vi "mod2.vi"() -> ()   [LabVIEW 2016]
doc: "\"Discrete LED demo.vi\" -- Demonstrate a discrete LED connected to a digital output.\n\nInstructions:\n\n-- Click the 'enable blinker' button to toggle between blinking mode\nand static mode.\n-- In static mode, click the 'digital level' button to set the state of the\ndigital output.\n-- The 'digital output state' LED indicator shows the state of the\ndigital output (on = high, off = low)."
uses:
  <vilib>/myRIO/Common/Instrument Driver Framework/myRIO v1.0/UART/vis/myRIO v1.0 Close UART.vi
  <vilib>/Utility/error.llb/Error Cluster From Error Code.vi
  <vilib>/myRIO/Common/Instrument Driver Framework/myRIO v1.0/DIO/vis/myRIO v1.0 Write DIO.vi
  <vilib>/myRIO/Common/Instrument Driver Framework/Utilities/vis/FPGA Ref Manager.vi
  <vilib>/myRIO/Common/Instrument Driver Framework/myRIO v1.0/myRIO v1.0 Reset FPGA.vi
  <vilib>/myRIO/Common/Instrument Driver Framework/myRIO v1.0/IRQ/vis/myRIO v1.0 IRQ Info FGV.vi
  <vilib>/myRIO/Common/Instrument Driver Framework/myRIO v1.0/IRQ/vis/myRIO v1.0 Timer IRQ Info FGV.vi
  <vilib>/myRIO/Common/Instrument Driver Framework/myRIO v1.0/IRQ/vis/myRIO v1.0 ISR Agent.vi
  <vilib>/myRIO/Instrument Drivers/Utilities/Utilities.lvlib
  <vilib>/myRIO/Instrument Drivers/Onboard IO/DIO/DIO.lvlib
panel:
  in  "String":string
  out "error out":errorcluster
  in  "error in (no error)":errorcluster
  in  "[ESC]":bool
  # "7-Segment LED demo"
  # "segment 'a'"
  # "segment 'b'"
  # "segment 'c'"
  # "segment 'd'"
  # "segment 'e'"
  # "segment 'f'"
  # "segment 'g'"
  # "decimal point"
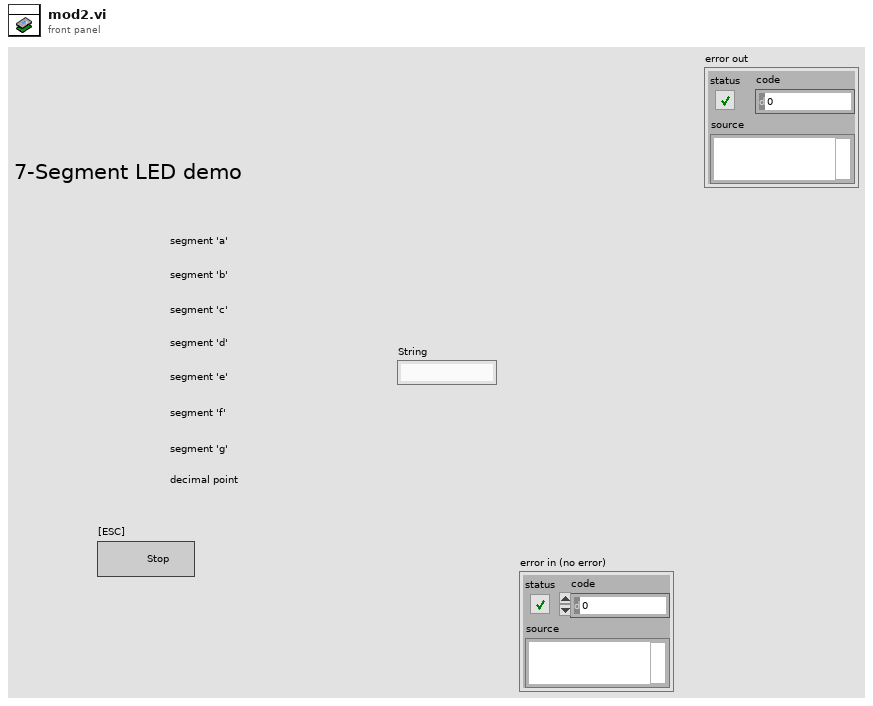
[diagram p1: front panel]
types:
  T1 = typedef "DIO.lvlib/DIO Reference.ctl" = cluster{"myRIO Reference":T2, "DIO Channels List":T6}
  T2 = typedef "myRIO Generic Hardware Reference.ctl" = cluster{"myRIO Model":T3, "myRIO Hardware Reference":T4}
  T3 = typedef "Hardware Version Enum.ctl" = enum16{"Unknown", "myRIO-1900", "myRIO-1950", "roboRIO", "NI ELVIS RIO CM"}
  T4 = typedef "myRIO v1.0 Reference.ctl" = cluster{"Generic FPGA Reference":T5, "Allow multiple opens":bool}
  T5 = typedef "Generic FPGA Reference.ctl" = refnum<k20>
  T6 = typedef "DIO Channels List.ctl" = T7[]
  T7 = typedef "DIO Channels Enum.ctl" = enum16{"Not Connected", "C/DIO0", "C/DIO1", "C/DIO2", "C/DIO3", "C/DIO4", "C/DIO5", "C/DIO6", "C/DIO7", "A/DIO0", "A/DIO1", "A/DIO2", "A/DIO3", "A/DIO4", "A/DIO5", "A/DIO6", "A/DIO7", "A/DIO8", "A/DIO9", "A/DIO10", "A/DIO11", "A/DIO12", "A/DIO13", "A/DIO14", "A/DIO15", "B/DIO0", "B/DIO1", "B/DIO2", "B/DIO3", "B/DIO4", "B/DIO5", "B/DIO6", "B/DIO7", "B/DIO8", "B/DIO9", "B/DIO10", "B/DIO11", "B/DIO12", "B/DIO13", "B/DIO14", "B/DIO15", "LED0", "LED1", "LED2", "LED3", "Button0", "DIO/DIO0", "DIO/DIO1", "DIO/DIO2", "DIO/DIO3", "DIO/DIO4", "DIO/DIO5", "DIO/DIO6", "DIO/DIO7", "DIO/DIO8", "DIO/DIO9", "SPI/CS0", "SPI/CS1", "SPI/CS2", "SPI/CS3", "LED RADIO (Green)", "LED RADIO (Red)", "LED COMM (Green)", "LED COMM (Red)", "LED MODE (Green)", "LED MODE (Red)"}
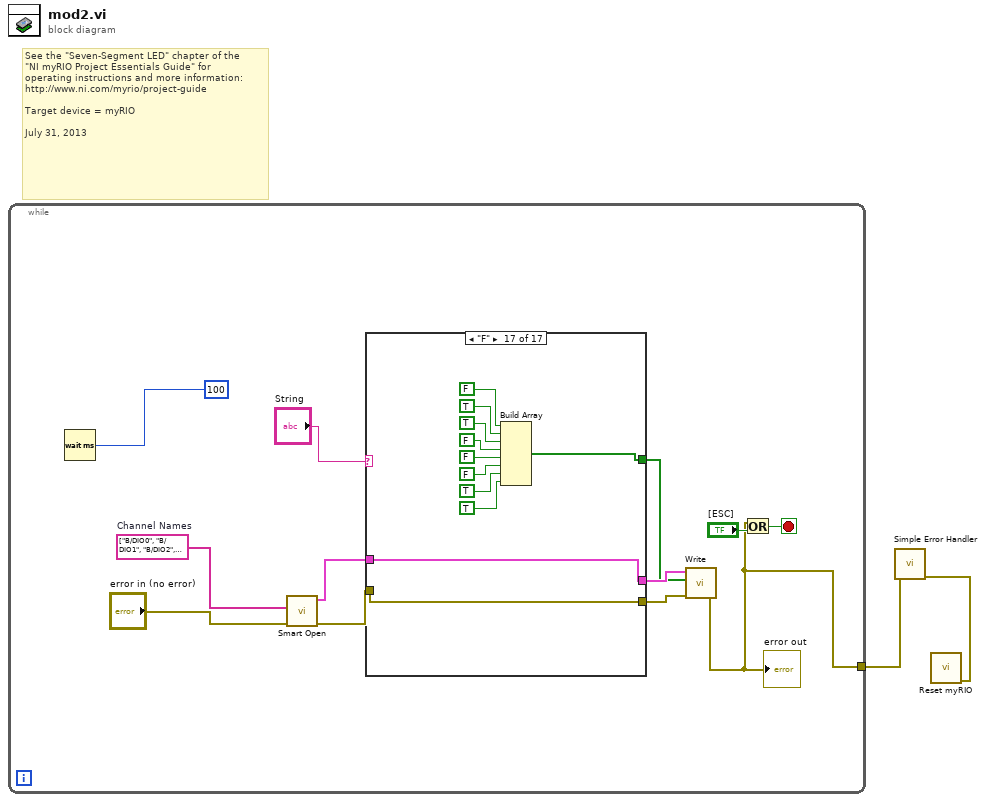
[diagram p0: block diagram]
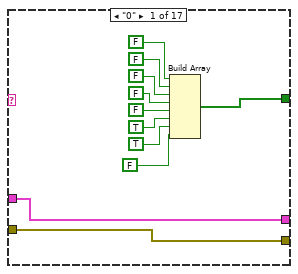
[diagram p2: hidden frame]
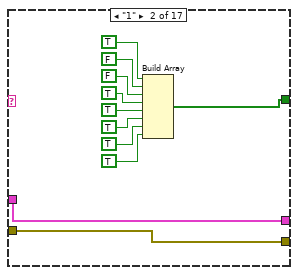
[diagram p3: hidden frame]
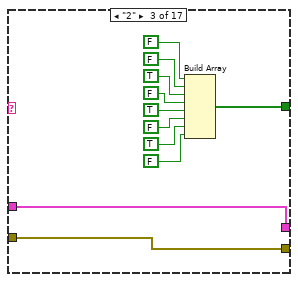
[diagram p4: hidden frame]
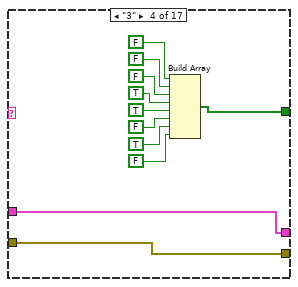
[diagram p5: hidden frame]
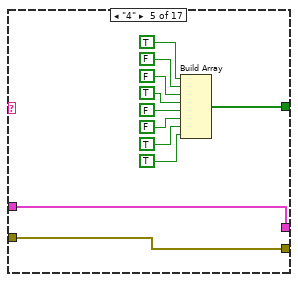
[diagram p6: hidden frame]
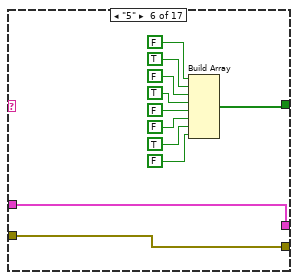
[diagram p7: hidden frame]
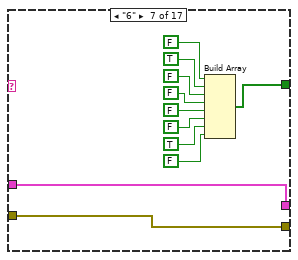
[diagram p8: hidden frame]
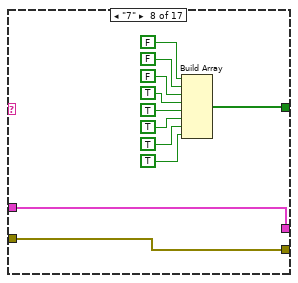
[diagram p9: hidden frame]
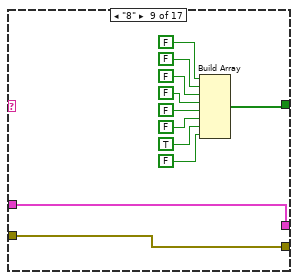
[diagram p10: hidden frame]
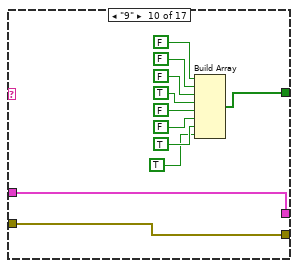
[diagram p11: hidden frame]
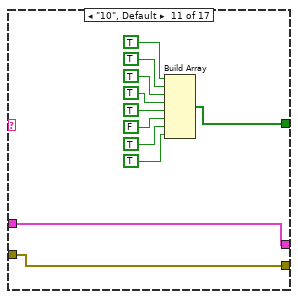
[diagram p12: hidden frame]
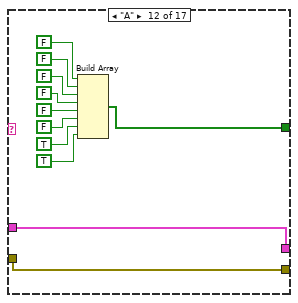
[diagram p13: hidden frame]
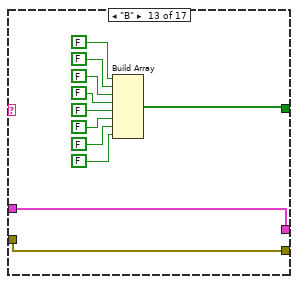
[diagram p14: hidden frame]
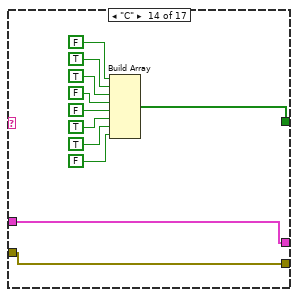
[diagram p15: hidden frame]
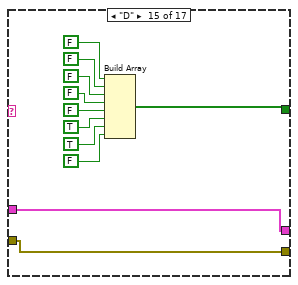
[diagram p16: hidden frame]
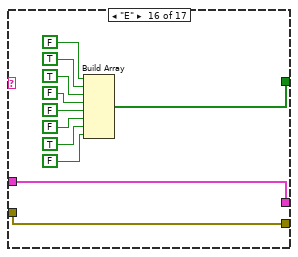
[diagram p17: hidden frame]
diagram:
  # "See the \"Seven-Segment LED\" chapter of the\n\"NI myRIO Project Essentials Guide\" for\noperating instructions and more information: \nhttp://www.ni.com/myrio/project-guide\n\nTarget device = myRIO\n\nJuly 31, 2013"
  n1 = while {
    tunnel: [w4] -> w2
    stop <- w9 stop-if-true
    w12 = tag[] ["B/DIO0", "B/DIO1", "B/DIO2", "B/DIO3", "B/DIO4", "B/DIO5", "B/DIO6", "B/DIO7"]  # Channel Names
    n2 = Wait (ms)(milliseconds to wait=u32 100) -> ()  [unwired: 1 out]
    n3 = call <vilib>:"Smart Open.vi"("error in (no error)"="error in (no error)", "Channel Names"=w12) -> ("error out"=w3:errorcluster, "DIO Ref Out"=w8:T1)  [unwired: 8 in]
    n4 = case shown="\"F\"" "String" {
      tunnel: w8 -> [w18 w28 w40 w51 w62 w73 w84 w95 w106 w117 w128 w137 w148 w159 w170 w181 w192]
      tunnel: [w18 w28 w40 w51 w62 w73 w84 w95 w106 w117 w128 w137 w148 w159 w170 w181 w192] -> w7
      tunnel: [w17 w27 w39 w50 w61 w72 w83 w94 w105 w116 w127 w136 w147 w158 w169 w180 w191] -> w6
      tunnel: [w16 w26 w38 w48 w60 w71 w82 w93 w104 w115 w125 w138 w149 w160 w171 w182 w193] -> w5
      tunnel: w3 -> [w17 w27 w39 w50 w61 w72 w83 w94 w105 w116 w127 w136 w147 w158 w169 w180 w191]
      frame "0" {
        n5 = Build Array(FALSE, FALSE, FALSE, FALSE, FALSE, TRUE, TRUE, FALSE) -> (w16:bool[])
      }
      frame "1" {
        n6 = Build Array(TRUE, FALSE, FALSE, TRUE, TRUE, TRUE, TRUE, TRUE) -> (w26:bool[])
      }
      frame "2" {
        n7 = Build Array(FALSE, FALSE, TRUE, FALSE, TRUE, FALSE, TRUE, FALSE) -> (w38:bool[])
      }
      frame "3" {
        n8 = Build Array(FALSE, FALSE, FALSE, TRUE, TRUE, FALSE, TRUE, FALSE) -> (w48:bool[])
      }
      frame "4" {
        n9 = Build Array(TRUE, FALSE, FALSE, TRUE, FALSE, FALSE, TRUE, TRUE) -> (w60:bool[])
      }
      frame "5" {
        n10 = Build Array(FALSE, TRUE, FALSE, TRUE, FALSE, FALSE, TRUE, FALSE) -> (w71:bool[])
      }
      frame "6" {
        n11 = Build Array(FALSE, TRUE, FALSE, FALSE, FALSE, FALSE, TRUE, FALSE) -> (w82:bool[])
      }
      frame "7" {
        n12 = Build Array(FALSE, FALSE, FALSE, TRUE, TRUE, TRUE, TRUE, TRUE) -> (w93:bool[])
      }
      frame "8" {
        n13 = Build Array(FALSE, FALSE, FALSE, FALSE, FALSE, FALSE, TRUE, FALSE) -> (w104:bool[])
      }
      frame "9" {
        n14 = Build Array(FALSE, FALSE, FALSE, TRUE, FALSE, FALSE, TRUE, TRUE) -> (w115:bool[])
      }
      frame "10", Default {
        n15 = Build Array(TRUE, TRUE, TRUE, TRUE, TRUE, FALSE, TRUE, TRUE) -> (w125:bool[])
      }
      frame "A" {
        n16 = Build Array(FALSE, FALSE, FALSE, FALSE, FALSE, FALSE, TRUE, TRUE) -> (w138:bool[])
      }
      frame "B" {
        n17 = Build Array(FALSE, FALSE, FALSE, FALSE, FALSE, FALSE, FALSE, FALSE) -> (w149:bool[])
      }
      frame "C" {
        n18 = Build Array(FALSE, TRUE, TRUE, FALSE, FALSE, TRUE, TRUE, FALSE) -> (w160:bool[])
      }
      frame "D" {
        n19 = Build Array(FALSE, FALSE, FALSE, FALSE, FALSE, TRUE, TRUE, FALSE) -> (w171:bool[])
      }
      frame "E" {
        n20 = Build Array(FALSE, TRUE, TRUE, FALSE, FALSE, FALSE, TRUE, FALSE) -> (w182:bool[])
      }
      frame "F" {
        n21 = Build Array(FALSE, TRUE, TRUE, FALSE, FALSE, FALSE, TRUE, TRUE) -> (w193:bool[])
      }
    }
    n22 = call <vilib>:"Write.vi"("error in (no error)"=w6, "Values"=w5, "DIO Ref In"=w7) -> ("error out"=w4:errorcluster)  [unwired: 6 in, 1 out]
    "error out" <- w4
    n23 = Or(x=w4, y="[ESC]") -> (x .or. y?=w9:bool)
  }
  n24 = call <vilib>:"Simple Error Handler.vi"("error in (no error)"=w2) -> ("error out"=w1:errorcluster)  [unwired: 4 in, 4 out]
  n25 = call <vilib>:"Reset myRIO.vi"("error in (no error)"=w1) -> ()  [unwired: 10 in, 1 out]
